vi "CommandReceived.vi"(8 "error in (no error)":errorcluster, 10 "ParsedData":refnum<class "ParsedData.lvclass">, 11 "DataReceived":refnum<class "DataReceived.lvclass">) -> (0 "error out":errorcluster, 3 "CommandReceived":refnum<class "CommandReceived.lvclass">)   [LabVIEW 2022 SP3, in "Cli.lvlib" / "CommandReceived.lvclass"]
uses:
  CommandReceived.lvclass
  Tcp/DataReceived/DataReceived.lvclass
  ArgumentParser/Source/ParsedData/ParsedData.lvclass
  CommandReceived.lvclass/CommandReceived.ctl
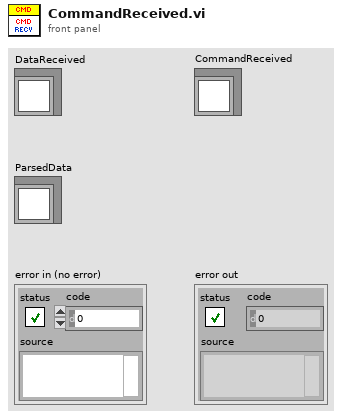
[diagram p1: front panel]
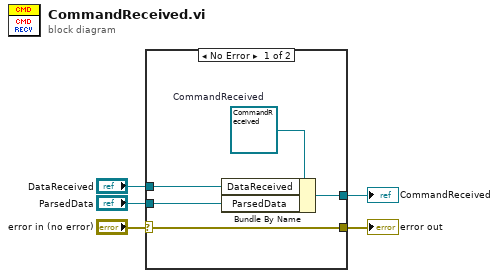
[diagram p0: block diagram]
diagram:
  n1 = case shown="No Error" "error in (no error)" {
    selector: "error in (no error)" -> [w10 w11]
    tunnel: [w10 w11] -> w4
    tunnel: [w8 _] -> w3
    tunnel: "ParsedData" -> [w7 _]
    tunnel: "DataReceived" -> [w6 _]
    frame No Error {
      w9 = refnum<class "CommandReceived.lvclass"> refnum  # CommandReceived
      n2 = Bundle By Name(cluster=w9, "DataReceived"=w6, "ParsedData"=w7) -> (w8:refnum<class "CommandReceived.lvclass">)
    }
    frame Error {
    }
  }
  "error out" <- w4
  "CommandReceived" <- w3
